vi "GotoZ.vi"(0 "Z Target Pos":sgl=-inf format="%#_g nm", 5 "error in":T1) -> (14 "Z Pos Out":sgl format="%#_g nm", 19 "error out":T1)   [LabVIEW 2016]
doc: "Changes the z position to the new value. By passing -Inf as input values, the current z position will be read out."
uses:
  Controls/Error_Out.ctl
  Files_ASC500/DLL/ASC500_RemoteControlV27.dll
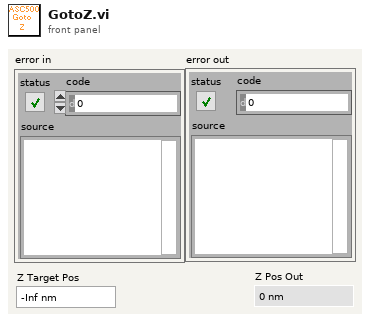
[diagram p1: front panel]
types:
  T1 = typedef "Error_Out.ctl" = errorcluster
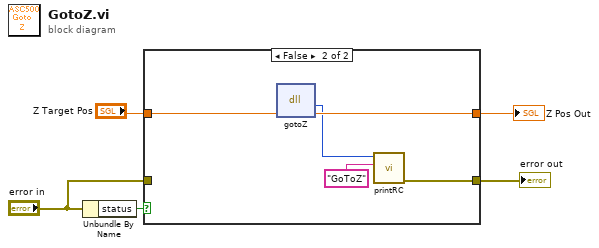
[diagram p0: block diagram]
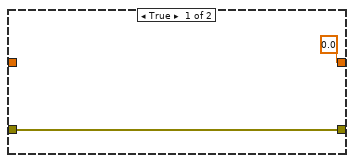
[diagram p2: hidden frame]
diagram:
  n1 = Unbundle By Name("error in") -> ("status"=w5:bool)
  n2 = case shown="False" w5 {
    tunnel: [w6 w9] -> w4
    tunnel: "Z Target Pos" -> [_ w12]
    tunnel: [sgl 0.0 ("Value") w11] -> w2
    tunnel: "error in" -> [w6 _]
    frame True {
    }
    frame False {
      n3 = dll-call lib="G:/SCMOperations/Share/ELE/Produkt Information/ASC500/04 Remote Control/02 development versions/2018Nov06/Files_ASC500/DLL/ASC500_RemoteControlV27.dll" fn="gotoZ"("Value"=w12) -> ("return type"=w10:i32, "Value"=w11:sgl)  [unwired: 3 in, 2 out]
      n4 = call "printRC.vi"("additional information"="GoToZ", "RC"=w10) -> ("error out"=w9:T1)  [unwired: 9 in]
    }
  }
  "error out" <- w4
  "Z Pos Out" <- w2
